vi "test3-SyncMessage_API.vi"(8 "error in (no error)":errorcluster, 11 "TestCase in":refnum<class "testcase-CSMMessage.lvclass">) -> (0 "error out":errorcluster, 3 "TestCase out":refnum<class "testcase-CSMMessage.lvclass">)   [LabVIEW 2017, in "testcase-CSMMessage.lvclass"]
uses:
  testcase-CSMMessage.lvclass
  31aab9b4-27f2-4601-9b9c-9d12425ab602.vi
  src/user.lib/_NEVSTOP/Communicable State Machine(CSM)/AdvanceAPI/CSM - Make String Arguments Safe.vi
  src/user.lib/_NEVSTOP/Communicable State Machine(CSM)/AdvanceAPI/CSM - Keywords.vi
  CSM/Global-TestcaseCSM.vi
  <vilib>/addons/_JKI Toolkits/VI Tester/TestCase.llb/TestCase.lvclass
  src/user.lib/_NEVSTOP/Communicable State Machine(CSM)/Communicable State Machine.lvlib
  CSM/CSM-Testcase.lvlib
  C:/Program Files (x86)/National Instruments/LabVIEW 2017/vi.lib/addons/_JKI Toolkits/VI Tester/TestCase.llb/TestCase.lvclass
panel:
  out "GlobalVar":T1(array[cluster])
  out "Attribute":T1(array[cluster])
  out "Found":bool[](array[boolean])
  out "Loopcount":i32
  out "concatenated string":string
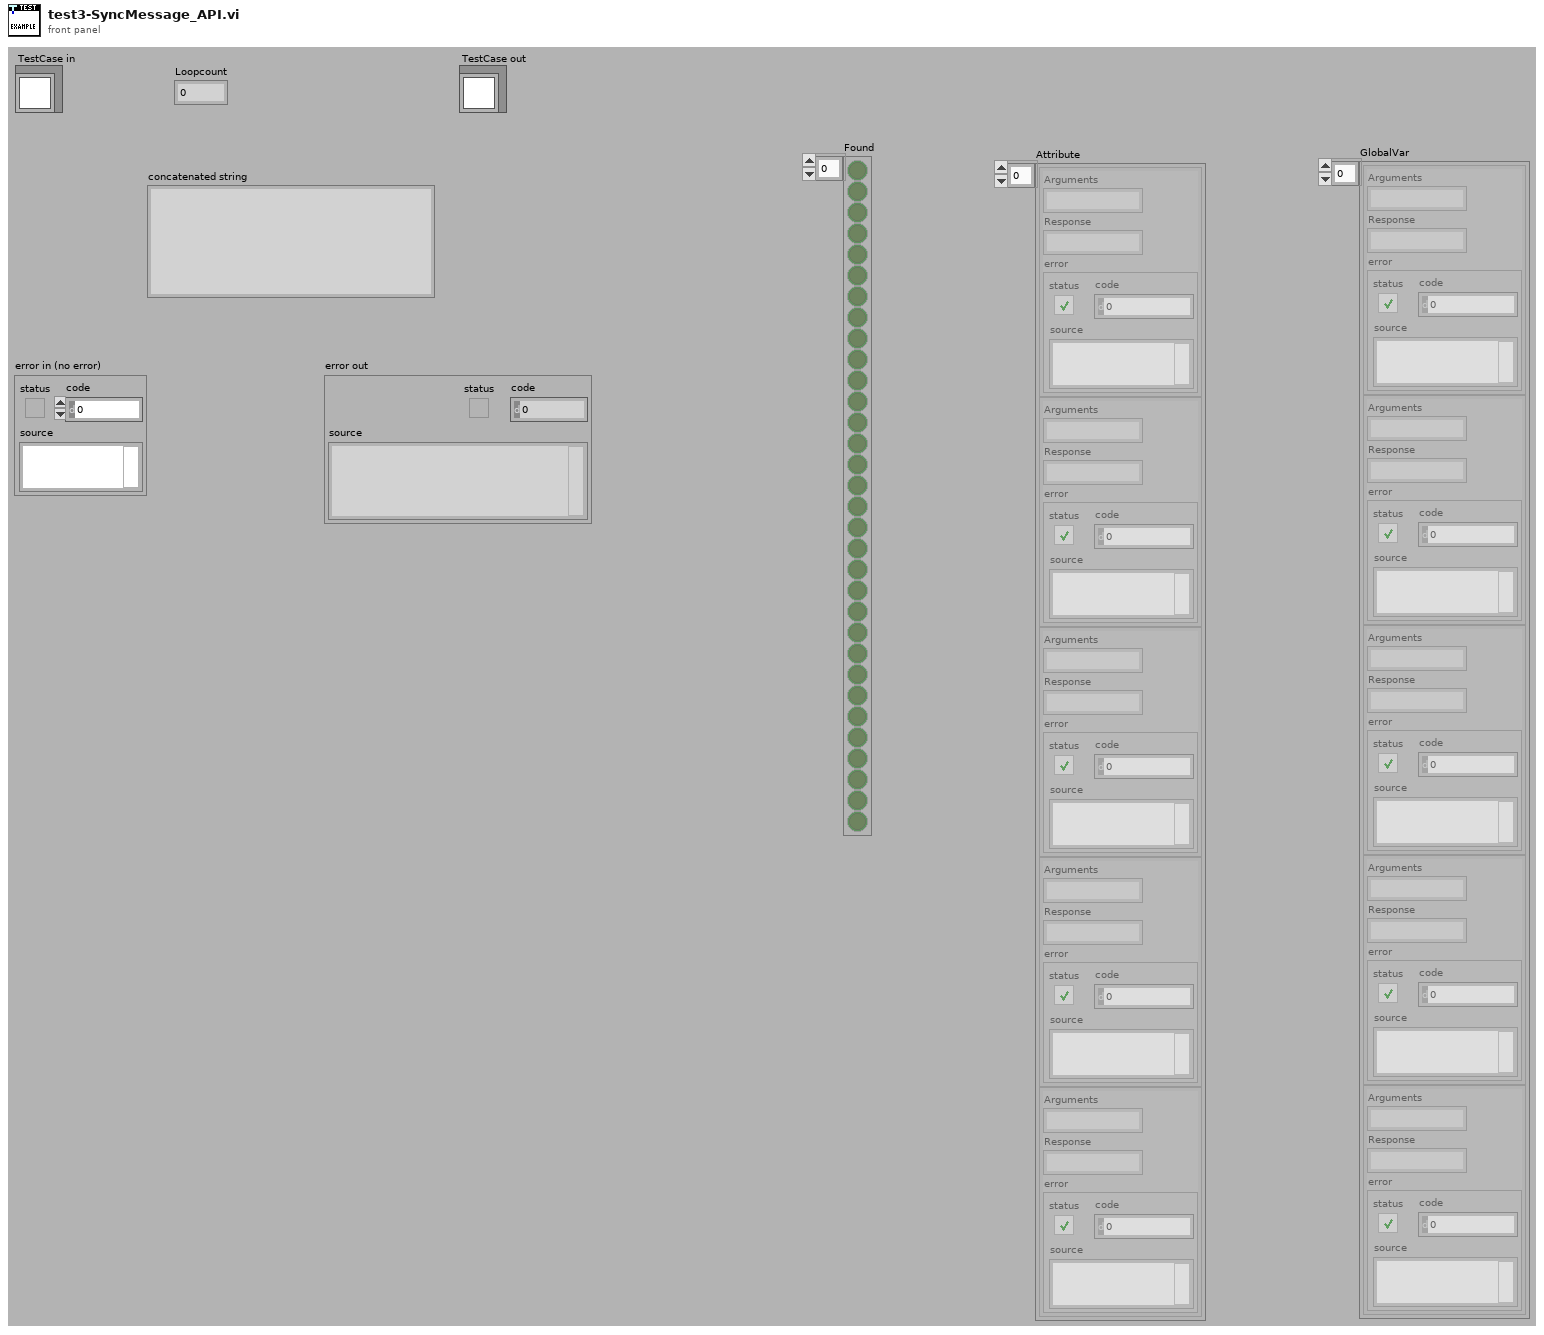
[diagram p1: front panel]
types:
  T1 = cluster{"Arguments":string, "Response":string, "error":errorcluster}[]
  T2 = cluster{"Arguments":string, "Response":string, "error":errorcluster}
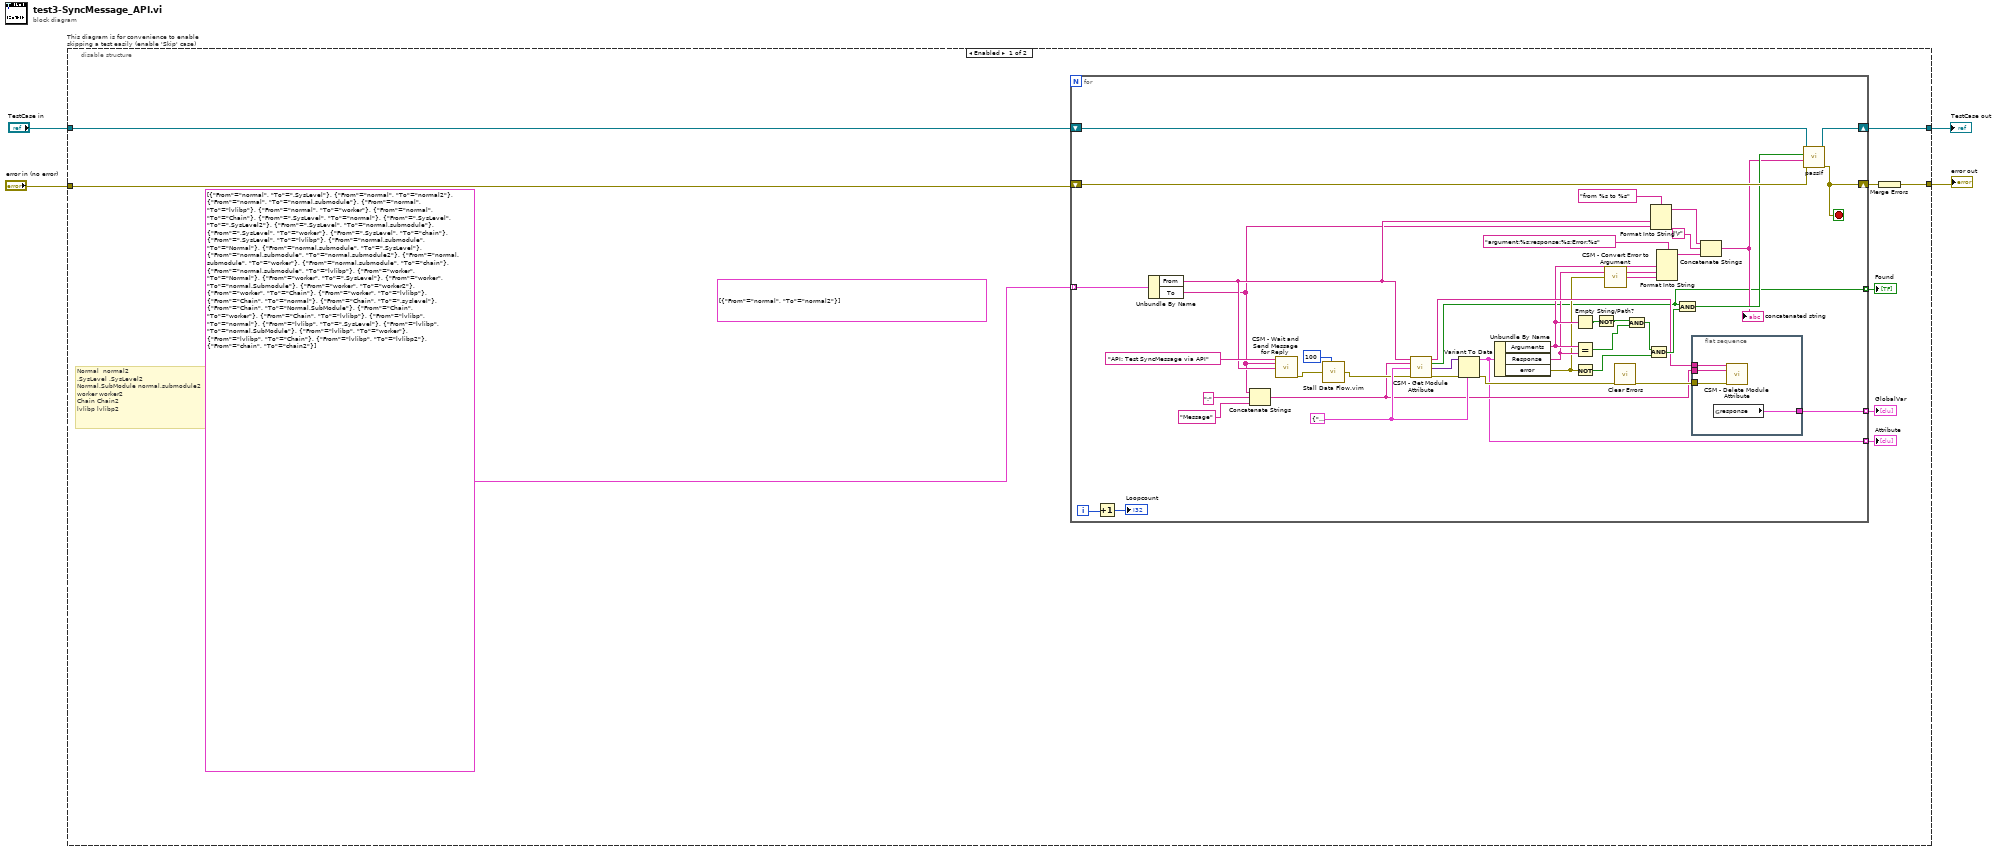
[diagram p0: block diagram]
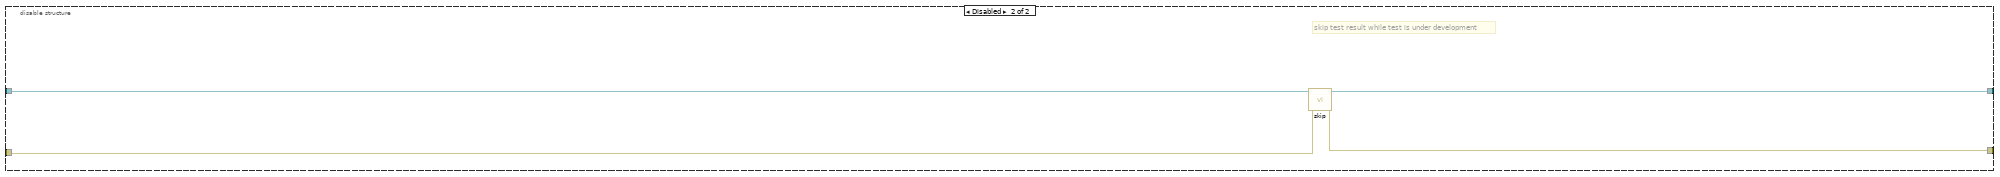
[diagram p2: hidden frame]
diagram:
  n1 = disable-structure "This diagram is for convenience to enable skipping a test easily (enable 'Skip' case)" shown="Enabled" {
    disable-tunnel: "TestCase in" -> [w13 w63]
    disable-tunnel: [w12 w61] -> w1
    disable-tunnel: [w9 w62] -> w3
    disable-tunnel: "error in (no error)" -> [w10 w60]
    frame Enabled {
      (unwired) cluster{"From":string, "To":string}[] [{"From"="normal", "To"="normal2"}]
      # "Normal  normal2\n.SysLevel .SysLevel2\nNormal.SubModule normal.submodule2\nworker worker2\nChain Chain2\nlvlibp lvlibp2"
      n2 = for {
        tunnel: cluster{"From":string, "To":string}[] [{"From"="normal", "To"=".SysLevel"}, {"From"="normal", "To"="normal2"}, {"From"="normal", "To"="normal.submodule"}, {"From"="normal", "To"="lvlibp"}, {"From"="normal", "To"="worker"}, {"From"="normal", "To"="Chain"}, {"From"=".SysLevel", "To"="normal"}, {"From"=".SysLevel", "To"=".SysLevel2"}, {"From"=".SysLevel", "To"="normal.submodule"}, {"From"=".SysLevel", "To"="worker"}, {"From"=".SysLevel", "To"="chain"}, {"From"=".SysLevel", "To"="lvlibp"}, {"From"="normal.submodule", "To"="Normal"}, {"From"="normal.submodule", "To"=".SysLevel"}, {"From"="normal.submodule", "To"="normal.submodule2"}, {"From"="normal.submodule", "To"="worker"}, {"From"="normal.submodule", "To"="chain"}, {"From"="normal.submodule", "To"="lvlibp"}, {"From"="worker", "To"="Normal"}, {"From"="worker", "To"=".SysLevel"}, {"From"="worker", "To"="normal.Submodule"}, {"From"="worker", "To"="worker2"}, {"From"="worker", "To"="Chain"}, {"From"="worker", "To"="lvlibp"}, {"From"="Chain", "To"="normal"}, {"From"="Chain", "To"=".syslevel"}, {"From"="Chain", "To"="Normal.SubModule"}, {"From"="Chain", "To"="worker"}, {"From"="Chain", "To"="lvlibp"}, {"From"="lvlibp", "To"="normal"}, {"From"="lvlibp", "To"=".SysLevel"}, {"From"="lvlibp", "To"="normal.SubModule"}, {"From"="lvlibp", "To"="worker"}, {"From"="lvlibp", "To"="Chain"}, {"From"="lvlibp", "To"="lvlibp2"}, {"From"="chain", "To"="chain2"}] -> [w46] mode=indexing
        shift-right: [w54] -> w12
        shift-left: w13 -> [w55]
        shift-right: [w27] -> w11
        shift-left: w10 -> [w53]
        tunnel: [w18] -> w7 mode=indexing
        tunnel: [w17] -> w6 mode=indexing
        tunnel: [w16] -> w5 mode=indexing
        i -> [w20]
        stop <- w27 stop-if-true
        w50 = T2 {"Arguments"="", "Response"="", "error"={"status"=FALSE, "code"=0, "source"=""}}
        n3 = Increment(x=w20) -> (x+1=→"Loopcount":i32)
        n4 = Unbundle By Name(w46) -> ("From"=w24:string, "To"=w22:string)
        n5 = Concatenate Strings(w22, ":" ("string"), "Message" ("string")) -> (w23:string)
        n6 = call "CSM - Wait and Send Message for Reply.vi"("State"="API: Test SyncMessage via API", "Arguments (\"\")"=w22, "Target Module"=w24) -> ("error out"=w15:errorcluster)  [unwired: 10 in, 2 out]
        n7 = call "Stall Data Flow.vim"("value in"=w15, "milliseconds to wait"=u32 100) -> ("value out"=w33:errorcluster)  [unwired: 1 out]
        n8 = call "CSM - Get Module Attribute.vi"("CSM Name"=w24, "Attribute"=w23, "Default Value (Empty Variant)"=w50, "Error In"=w33) -> ("CSM Name (Dup)"=w44:string, "Found"=w18:bool, "Value"=w21:variant, "error out"=w51:errorcluster)  [unwired: 7 in, 1 out]
        n9 = Variant To Data(error in=w51, type=w50, Variant=w21) -> (data=w17:T2, error out=w29:errorcluster)
        n10 = Unbundle By Name(w17) -> ("Arguments"=w39:string, "Response"=w38:string, "error"=w36:errorcluster)
        n11 = Empty String/Path?(string/path=w39) -> (empty?=w43:bool)
        n12 = Equal?(x=w39, y=w38) -> (x = y?=w41:bool)
        n13 = Not(x=w36) -> (.not. x?=w49:bool)
        n14 = Not(x=w43) -> (.not. x?=w42:bool)
        n15 = call "CSM - Convert Error to Argument.vi"("Error"=w36) -> ("Argument"=w37:string)  [unwired: 4 in]
        n16 = call <vilib>:"Clear Errors.vi"("error in (no error)"=w29) -> ("error out"=w28:errorcluster)  [unwired: 5 in, 1 out]
        n17 = And(x=w42, y=w41) -> (x .and. y?=w40:bool)
        n18 = And(x=w40, y=w49) -> (x .and. y?=w48:bool)
        n19 = Format Into String(format string="from %s to %s", w24, w22) -> (resulting string=w31:string)  [unwired: 2 in, 1 out]
        n20 = Format Into String(format string="argument:%s;response:%s;Error:%s", w39, w38, w37) -> (resulting string=w35:string)  [unwired: 2 in, 1 out]
        n21 = And(x=w18, y=w48) -> (x .and. y?=w47:bool)
        n22 = flat-sequence {
          tunnel: w44 -> [w59]
          tunnel: w28 -> [w58]
          tunnel: w23 -> [w57]
          tunnel: [w56] -> w16
          frame #0 {
            n23 = global read "Global-TestcaseCSM.vi" "response"() -> (w56:T2)
            n24 = call "CSM - Delete Module Attribute.vi"("CSM Name"=w59, "Attribute"=w57, "Error In"=w58) -> ()  [unwired: 9 in, 4 out]
          }
        }
        n25 = Concatenate Strings(w31, "\r", w35) -> (w32:string)
        "concatenated string" <- w32
        n26 = call-dynamic "passIf.vi"("error in (no error)"=w53, "message (\"\")"=w32, "pass"=w47, "TestCase in"=w55) -> ("error out"=w27:errorcluster, "TestCase out"=w54:refnum<class "testcase-CSMMessage.lvclass">)  [unwired: 6 in]
      }
      "Found" <- w7
      "Attribute" <- w6
      "GlobalVar" <- w5
      n27 = Merge Errors(w11) -> (w9:errorcluster)
    }
    frame Disabled {
      # "skip test result while test is under development"
      n28 = call <vilib>:"skip.vi"("error in (no error)"=w60, "TestCase in"=w63) -> ("error out"=w62:errorcluster, "TestCase out"=w61:refnum<class "testcase-CSMMessage.lvclass">)  [unwired: 8 in]
    }
  }
  "error out" <- w3
  "TestCase out" <- w1
